vi "ILD1420_Global.vi"() -> ()   [LabVIEW 2015]
panel:
  in  "ILD1420 COM port":refnum<visa-resource-name>
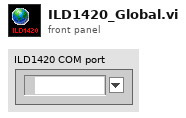
[diagram p1: front panel]
diagram:
